vi "Set LED Color.vi"(0 "Session In":refnum<visa-resource-name>, 5 "Red":dbl(slide) scale=0.0..1.0, 7 "Green":dbl(slide) scale=0.0..1.0, 9 "Blue":dbl(slide) scale=0.0..1.0, 11 "error in":errorcluster {"code" format="%.0x"}) -> (4 "Session Out":refnum<visa-resource-name>, 15 "error out":errorcluster {"code" format="%.0x"})   [LabVIEW 2012, in "YOST 3 Space.lvlib"]
uses:
  YOST 3 Space.lvlib
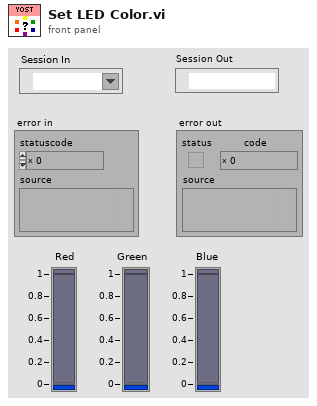
[diagram p1: front panel]
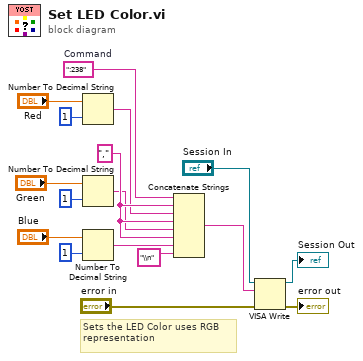
[diagram p0: block diagram]
diagram:
  w12 = "," ("string")
  w15 = ":238"  # Command
  # "Sets the LED Color uses RGB representation"
  n1 = Number To Decimal String(number="Red", width (-)=i16 1) -> (decimal integer string=w3:string)
  n2 = Number To Decimal String(number="Green", width (-)=i16 1) -> (decimal integer string=w9:string)
  n3 = Number To Decimal String(number="Blue", width (-)=i16 1) -> (decimal integer string=w1:string)
  n4 = Concatenate Strings(w15, w12, w3, w12, w9, w12, w1, "\\n" ("string")) -> (w14:string)
  n5 = VISA Write(VISA resource name="Session In", write buffer=w14, error in (no error)="error in") -> (VISA resource name out=→"Session Out":refnum<visa-resource-name>, error out=→"error out":errorcluster)  [unwired: 1 out]
